vi "Tosca-Start 2P.vi"(0 "Tosca":refnum<class "Parameters.lvclass">, 11 "error in (no error)":errorcluster) -> (4 "Tosca out":refnum<class "Parameters.lvclass">, 15 "error out":errorcluster)   [LabVIEW 2020]
uses:
  Classes/Parameters/Parameters.lvclass
  Classes/Parameters/Parameters.lvclass/Parameters.ctl
  Classes/Parameters/Read Imaging.vi
  Classes/Parameters/Read DAQ.vi
  Classes/Parameters/Read mode.vi
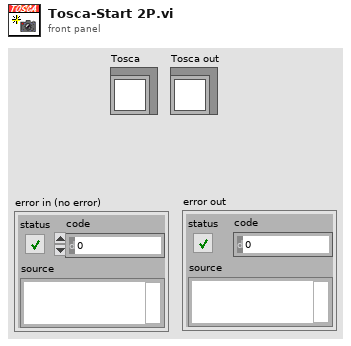
[diagram p1: front panel]
types:
  T1 = typedef "Tosca-Imaging.ctl" = cluster{"mode":T2, "FrameRateHz":dbl, "use AO":bool, "destination":string}
  T2 = typedef "Tosca-Imaging Mode.ctl" = enum16{"Off", "Widefield", "Two-photon"}
  T3 = typedef "Parameters.lvclass/DAQ.ctl" = cluster{"AO Fs (Hz)":dbl, "DO Fs (Hz)":dbl, "Poll Rate (Hz)":dbl, "Baseline (s)":dbl}
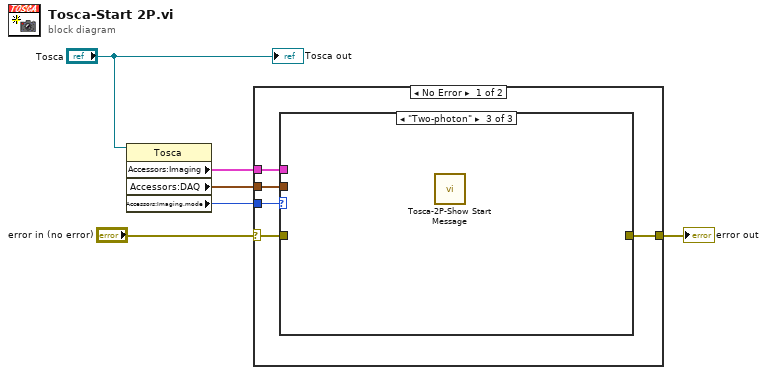
[diagram p0: block diagram]
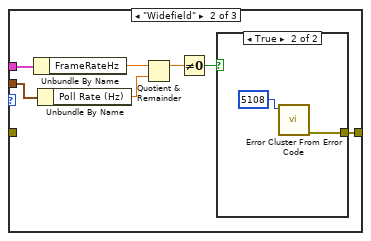
[diagram p3: hidden frame]
diagram:
  n1 = property class="Tosca"(reference="Tosca") -> ("Accessors:Imaging"=w2:T1, "Accessors:DAQ"=w1:T3, "Accessors:Imaging.mode"=w3:T2)  [unwired: 1 in, 2 out]
  n2 = case shown="No Error" "error in (no error)" {
    selector: "error in (no error)" -> [w10 w22]
    tunnel: [w11 w22] -> w6
    tunnel: w3 -> [w9 _]
    tunnel: w2 -> [w8 _]
    tunnel: w1 -> [w7 _]
    frame No Error {
      n3 = case shown="\"Two-photon\"" w9 {
        tunnel: [w12 w16 _] -> w11
        tunnel: w10 -> [w12 _ _]
        tunnel: w8 -> [_ w15 _]
        tunnel: w7 -> [_ w14 _]
        frame "Off", Default {
        }
        frame "Widefield" {
          n4 = Unbundle By Name(w15) -> ("FrameRateHz"=w17:dbl)
          n5 = Unbundle By Name(w14) -> ("Poll Rate (Hz)"=w13:dbl)
          n6 = Quotient & Remainder(x=w17, y=w13) -> (x-y*floor(x/y)=w19:dbl)  [unwired: 1 out]
          n7 = Not Equal To 0?(x=w19) -> (x != 0?=w18:bool)
          n8 = case shown="True" w18 {
            tunnel: [_ w20] -> w16
            frame False {
            }
            frame True {
              n9 = call <vilib>:"Error Cluster From Error Code.vi"("error code (0)"=5108) -> ("error out"=w20:errorcluster)  [unwired: 8 in]
            }
          }
        }
        frame "Two-photon" {
          n10 = call "Tosca-2P-Show Start Message.vi"() -> ()  [unwired: 16 in]
        }
      }
    }
    frame Error {
    }
  }
  "error out" <- w6
  "Tosca out" <- "Tosca"
